vi "Configure OAuth.vi"(4 "Grant Flow (PKCE)":T1=enum."Authorization Code (PKCE)", 5 "Oauth2 in":refnum<class "Oauth2.lvclass">, 6 "Refresh Token":string, 7 "Exchange Code Server URI":string caption="Exchange Code Server URI (empty: same as Auth Server)", 8 "scopes":string[](array[string]), 9 "Client Secret":string, 10 "Client ID":string, 11 "Authorization Server URI":string) -> (0 "error out":errorcluster, 3 "Oauth2":refnum<class "Oauth2.lvclass">)   [LabVIEW 2017, in "Oauth2.lvclass"]
doc: "Added Grant Flow enum as an input option.\n\nAllows for constructing a specific URI when a OAuth Server accepts multiple flows.\n\nAuthorization Code with PKCE is the preferred method."
uses:
  Oauth2.lvclass
  OAuth2 Flow -- enum.ctl
  OAuthToken/OAuth2 Token Element -- enum.ctl
  Oauth2.lvclass/Oauth2.ctl
  <vilib>/Utility/error.llb/Trim Whitespace One-Sided.vi
  OAuthToken/Retrieve Element.vi
  <vilib>/LabVIEW Open Source Project/OpenURI/uri/Get URI.vi
  <vilib>/LabVIEW Open Source Project/OpenURI/uri/URI.lvclass
  OAuthToken/OAuthAccessToken.lvclass
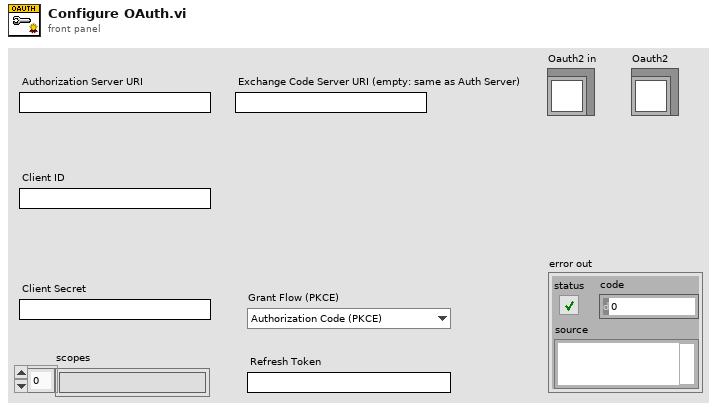
[diagram p1: front panel]
types:
  T1 = typedef "Oauth2.lvclass/OAuth2 Flow -- enum.ctl" = enum16{"Authorization Code", "Authorization Code (PKCE)", "Implicit", "Resource Owner Credentials", "Client Credentials", "Refresh Token", "Device Code"}
  T2 = typedef "OAuthAccessToken.lvclass/OAuth2 Token Element -- enum.ctl" = enum16{"client_id", "client_secret", "response_type", "scope", "redirect_uri", "error", "error_description", "error_uri", "grant_type", "code", "access_token", "token_type", "expires_in", "username", "password", "refresh_token", "code_challenge", "code_challenge_method", "reverse_proxy_uri", "endpoint element", "prompt", "access_type", "id_token"}
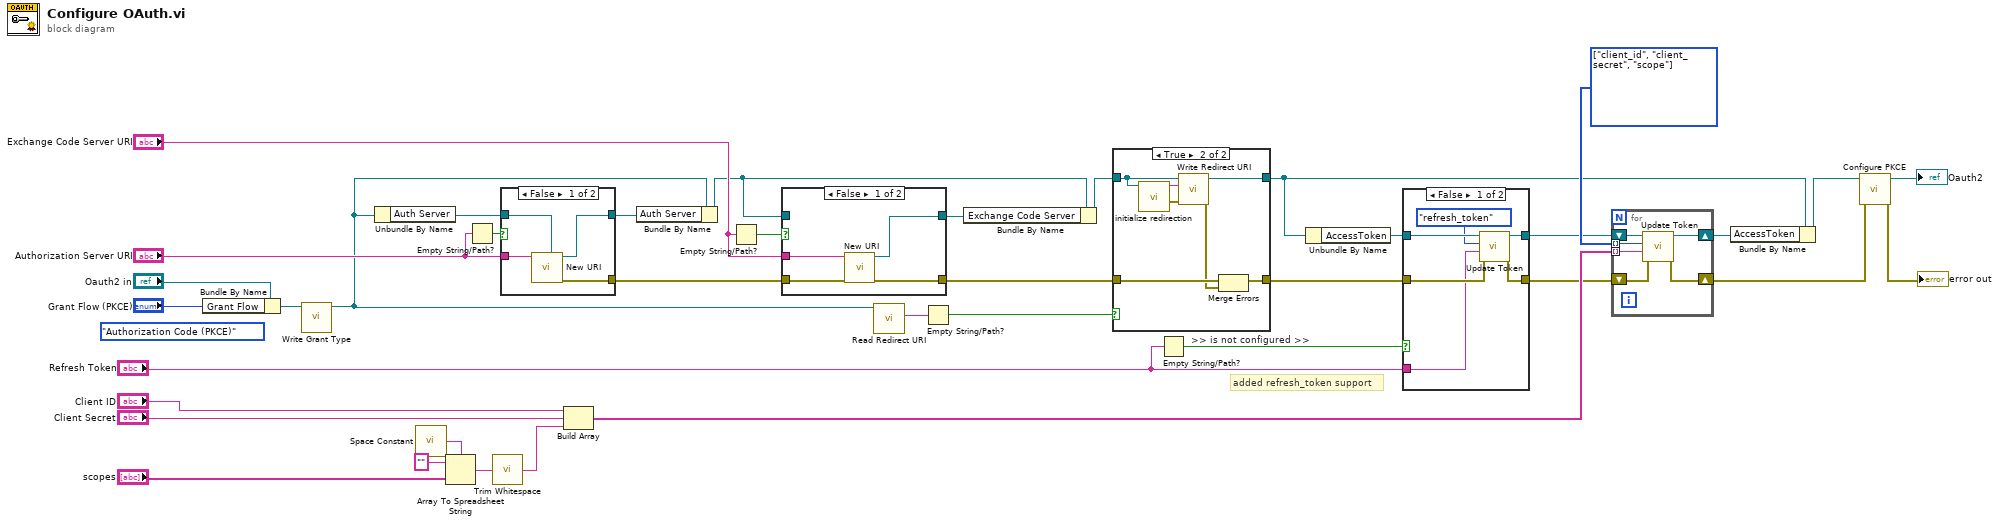
[diagram p0: block diagram]
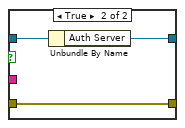
[diagram p3: hidden frame]
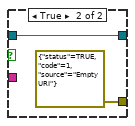
[diagram p4: hidden frame]
diagram:
  (unwired) OAuth2_Flow_--_enum."Authorization Code (PKCE)" ("Grant Flow (PKCE)")
  w29 = T2[] [enum."client_id", enum."client_secret", enum."scope"] items=["client_id", "client_secret", "response_type", "scope", "redirect_uri", "error", "error_description", "error_uri", "grant_type", "code", "access_token", "token_type", "expires_in", "username", "password", "refresh_token", "code_challenge", "code_challenge_method", "reverse_proxy_uri", "endpoint element", "prompt", "access_type", "id_token"]
  # "added refresh_token support"
  n1 = Bundle By Name(cluster="Oauth2 in", "Grant Flow"="Grant Flow (PKCE)") -> (w2:refnum<class "Oauth2.lvclass">)
  n2 = call-dynamic "Write Grant Type.vi"("Oauth2 in"=w2) -> ("Oauth2 out"=w1:refnum<class "Oauth2.lvclass">)  [unwired: 9 in, 1 out]
  n3 = Unbundle By Name(w1) -> ("Auth Server"=w38:refnum<class "URI.lvclass">)
  n4 = call <vilib>:"Space Constant.vi"() -> ("String"=w33:string)
  n5 = Array To Spreadsheet String(delimiter (Tab)=w33, array="scopes", 3:"" ("format string")) -> (spreadsheet string=w34:string)
  n6 = Empty String/Path?(string/path="Authorization Server URI") -> (empty?=w35:bool)
  n7 = call <vilib>:"Trim Whitespace.vi"("string"=w34) -> ("trimmed string"=w25:string)  [unwired: 1 in]
  n8 = case shown="False" w35 {
    tunnel: w38 -> [w42 w44]
    tunnel: [w41 w44] -> w37
    tunnel: "Authorization Server URI" -> [w40 _]
    tunnel: [w39 errorcluster {"status"=TRUE, "code"=1, "source"="Empty URI"} ("error out")] -> w17
    frame False {
      n9 = call <vilib>:"New URI.vi"("URI in"=w42, "URI"=w40) -> ("error out"=w39:errorcluster, "URI"=w41:refnum<class "URI.lvclass">)  [unwired: 8 in]
    }
    frame True {
    }
  }
  n10 = Build Array("Client ID", "Client Secret", w25) -> (w26:string[])
  n11 = Bundle By Name(cluster=w1, "Auth Server"=w37) -> (w11:refnum<class "Oauth2.lvclass">)
  n12 = Empty String/Path?(string/path="Exchange Code Server URI") -> (empty?=w15:bool)
  n13 = case shown="False" w15 {
    tunnel: [w48 w49] -> w13
    tunnel: "Exchange Code Server URI" -> [w47 _]
    tunnel: [w46 w51] -> w16
    tunnel: w17 -> [w45 w51]
    tunnel: w11 -> [_ w50]
    frame False {
      n14 = call <vilib>:"New URI.vi"("error in (no error)"=w45, "URI"=w47) -> ("error out"=w46:errorcluster, "URI"=w48:refnum<class "URI.lvclass">)  [unwired: 8 in]
    }
    frame True {
      n15 = Unbundle By Name(w50) -> ("Auth Server"=w49:refnum<class "URI.lvclass">)
    }
  }
  n16 = call "Read Redirect URI.vi"("Oauth2 in"=w1) -> ("Redirect URI"=w24:string)  [unwired: 8 in, 2 out]
  n17 = Empty String/Path?(string/path=w24) -> (empty?=w23:bool)
  n18 = Bundle By Name(cluster=w11, "Exchange Code Server"=w13) -> (w12:refnum<class "Oauth2.lvclass">)
  n19 = case shown="True" w23 {
    tunnel: w12 -> [w53 w57]
    tunnel: [w53 w60] -> w5
    tunnel: [w52 w55] -> w10
    tunnel: w16 -> [w52 w56]
    frame False {
    }
    frame True {
      n20 = call-dynamic "initialize redirection.vi"("Oauth2"=w57) -> ("error out"=w58:errorcluster, "Redirect URI"=w59:string)  [unwired: 9 in]
      n21 = call "Write Redirect URI.vi"("error in (no error)"=w58, "Redirect URI"=w59, "Oauth2 in"=w57) -> ("error out"=w54:errorcluster, "Oauth2 out"=w60:refnum<class "Oauth2.lvclass">)  [unwired: 7 in]
      n22 = Merge Errors(w56, w54) -> (w55:errorcluster)
    }
  }
  n23 = Empty String/Path? ">> is not configured >>"(string/path="Refresh Token") -> (empty?=w9:bool)
  n24 = Unbundle By Name(w5) -> ("AccessToken"=w7:refnum<class "OAuthAccessToken.lvclass">)
  n25 = case shown="False" w9 {
    tunnel: [w63 w67] -> w8
    tunnel: w10 -> [w64 w67]
    tunnel: w7 -> [w66 w68]
    tunnel: [w65 w68] -> w6
    tunnel: "Refresh Token" -> [w61 _]
    frame False {
      n26 = call "Update Token.vi"("error in (no error)"=w64, "Value"=w61, "Token element"=OAuth2_Token_Element_--_enum."refresh_token", "OAuthAccessToken in"=w66) -> ("error out"=w63:errorcluster, "OAuthAccessToken out"=w65:refnum<class "OAuthAccessToken.lvclass">)  [unwired: 6 in]
    }
    frame True {
    }
  }
  n27 = for {
    tunnel: w26 -> [w73] mode=indexing
    shift-right: [w72] -> w30
    shift-left: w6 -> [w74]
    tunnel: w29 -> [w71] mode=indexing
    shift-right: [w69] -> w19
    shift-left: w8 -> [w70]
    n28 = call "Update Token.vi"("error in (no error)"=w70, "Value"=w73, "Token element"=w71, "OAuthAccessToken in"=w74) -> ("error out"=w69:errorcluster, "OAuthAccessToken out"=w72:refnum<class "OAuthAccessToken.lvclass">)  [unwired: 6 in]
  }
  n29 = Bundle By Name(cluster=w5, "AccessToken"=w30) -> (w21:refnum<class "Oauth2.lvclass">)
  n30 = call "Configure PKCE.vi"("error in"=w19, "Oauth2 in"=w21) -> ("error out"=→"error out":errorcluster, "Oauth2"=→"Oauth2":refnum<class "Oauth2.lvclass">)  [unwired: 8 in]
